vi "Cleanup.vi"(8 "error in (no error)":errorcluster, 11 "Chat Server in":refnum<class "Chat Server.lvclass">) -> (0 "error out":errorcluster)   [LabVIEW 2020, in "Chat Server.lvclass"]
uses:
  Chat Server.lvclass
  Chat Server.lvclass/Chat Server.ctl
  Stream-TCP/TCP Server/TCP Server.lvclass
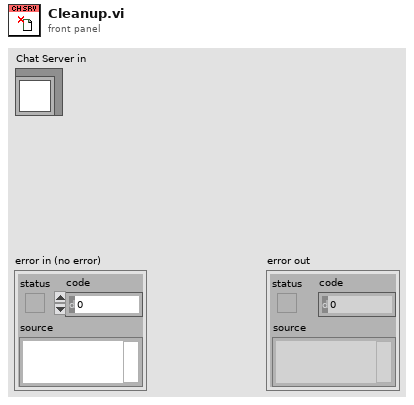
[diagram p1: front panel]
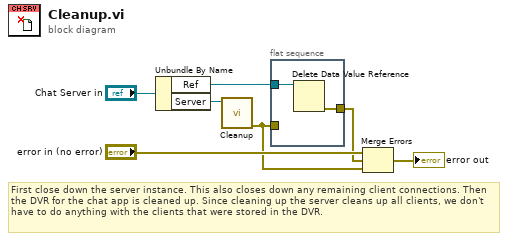
[diagram p0: block diagram]
diagram:
  # "First close down the server instance. This also closes down any remaining client connections. Then the DVR for the chat app is cleaned up. Since cleaning up the server cleans up all clients, we don't have to do anything with the clients that were stored in the DVR."
  n1 = Unbundle By Name("Chat Server in") -> ("Ref"=w4:refnum<data-value>, "Server"=w5:refnum<class "TCP Server.lvclass">)
  n2 = call-dynamic "Cleanup.vi"("TCP Server in"=w5) -> ("error out"=w2:errorcluster)  [unwired: 10 in]
  n3 = flat-sequence {
    tunnel: w4 -> [w9]
    tunnel: [w8] -> w1
    tunnel: w2 -> [_]
    frame #0 {
      n4 = Delete Data Value Reference(data value reference=w9) -> (error out=w8:errorcluster)  [unwired: 1 in, 1 out]
    }
  }
  n5 = Merge Errors("error in (no error)", w1, w2) -> (→"error out":errorcluster)
